vi "FTW-Endpoint-IncomingRequestProxy-Receive.vi"(0 "FTW ØMQ Endpoint":refnum<class "FTW-Endpoint-ZMQ.lvclass">, 11 "error in":errorcluster) -> (4 "FTW ØMQ Endpoint out":refnum<class "FTW-Endpoint-ZMQ.lvclass">, 6 "Message Received":string[](array[string]), 8 "Timed out?":bool, 15 "error out":errorcluster)   [LabVIEW 2012, in "FTW-Endpoint-ZMQ.lvclass"]
uses:
  FTW-Endpoint-ZMQ.lvclass
  FTW-Endpoint-ZMQ.lvclass/FTW-Endpoint-ZMQ.ctl
panel:
  # "Inputs"
  # "Outputs"
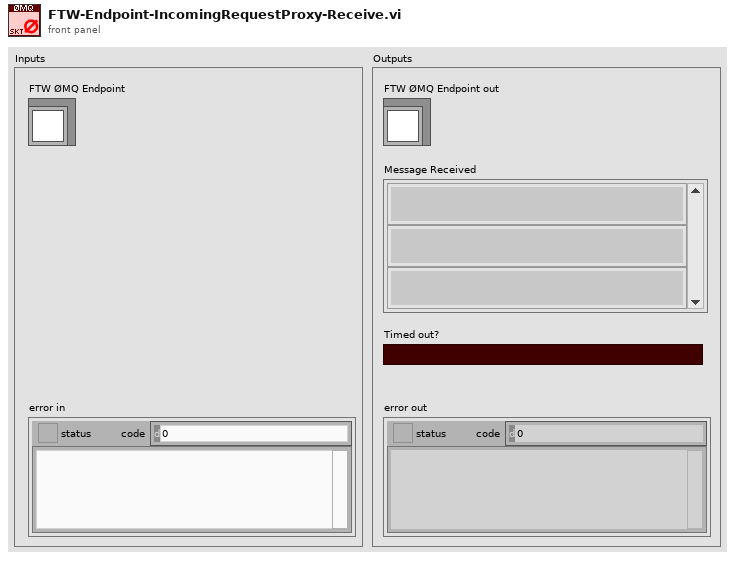
[diagram p1: front panel]
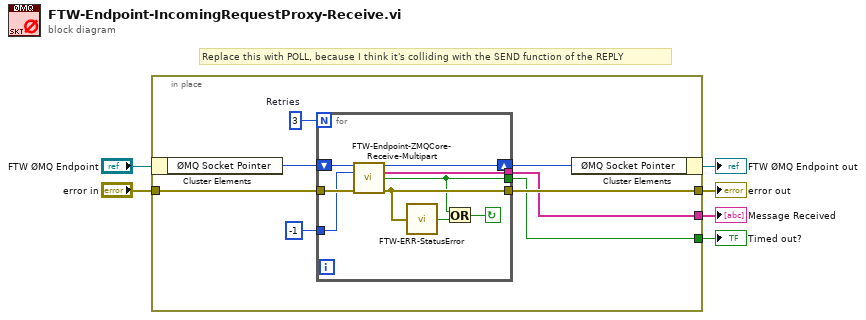
[diagram p0: block diagram]
diagram:
  # "Replace this with POLL, because I think it's colliding with the SEND function of the REPLY"
  n1 = in-place {
    in-place-border: [w11] -> w4
    in-place-border: [w12] -> w3
    in-place-border: "error in" -> [w13]
    in-place-border: [w9] -> w1
    w8 = 3  # Retries
    n2 = in-place-cluster #1("FTW ØMQ Endpoint") -> ("ØMQ Socket Pointer"=w14:u64)
    n3 = for {
      N: w8 -> [_]
      tunnel: w13 -> [w22]
      tunnel: [w19] -> w12
      tunnel: [w21] -> w11
      tunnel: [w16] -> w9
      shift-right: [w20] -> w10
      shift-left: w14 -> [w23]
      tunnel: -1 ("Timeout") -> [w15]
      stop <- w17 continue-if-true
      n4 = call "FTW-Endpoint-ZMQCore-Receive-Multipart.vi"("ØMQ Socket Pointer"=w23, "Timeout"=w15, "error in"=w22) -> ("ØMQ Socket Pointer out"=w20:u64, "Multipart Message"=w21:string[], "Timed out?"=w16:bool, "error out"=w19:errorcluster)  [unwired: 9 in]
      n5 = call "FTW-ERR-StatusError.vi"("error to check"=w19) -> ("Error?"=w18:bool)
      n6 = Or(x=w16, y=w18) -> (x .or. y?=w17:bool)
    }
    n7 = in-place-cluster #1("ØMQ Socket Pointer"=w10) -> (→"FTW ØMQ Endpoint out":refnum<class "FTW-Endpoint-ZMQ.lvclass">)
  }
  "error out" <- w3
  "Message Received" <- w4
  "Timed out?" <- w1
